vi "practica14RNA.vi"() -> ()   [LabVIEW 2016]
panel:
  out "XY Graph 2":cluster{dbl[], dbl[]}[](graph)
  out "axon":dbl
  in  "B":dbl
  in  "W2":dbl
  in  "W1":dbl
  in  "X2":dbl
  in  "X1":dbl
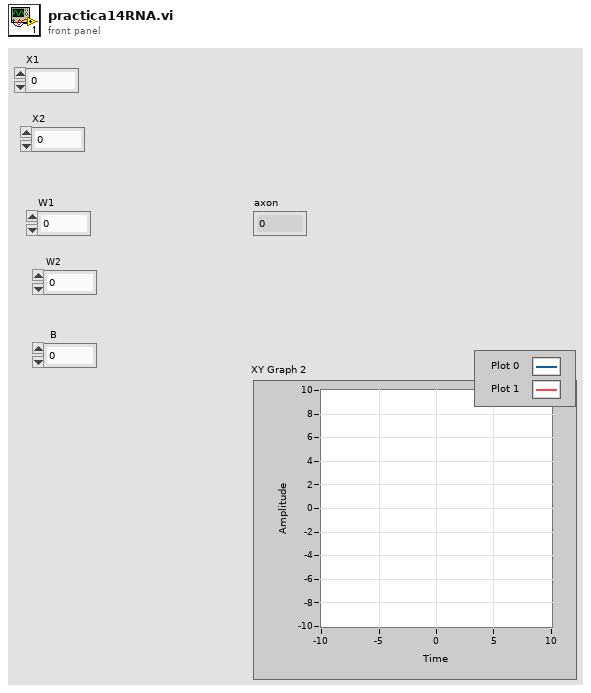
[diagram p1: front panel]
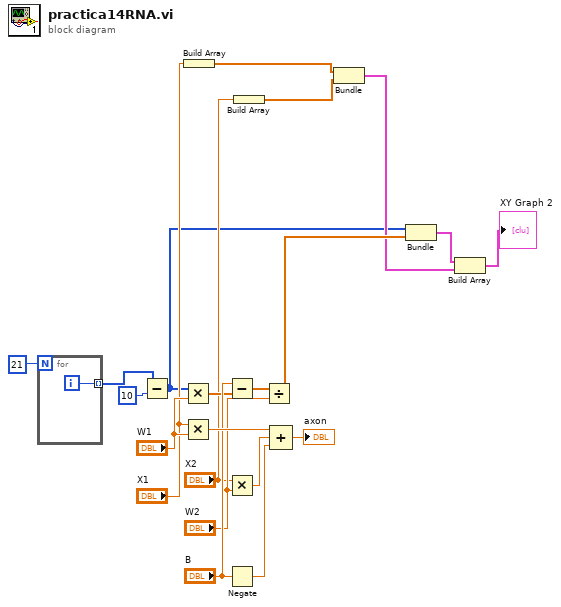
[diagram p0: block diagram]
diagram:
  n1 = for {
    N: 21 -> [_]
    tunnel: [w22] -> w2 mode=indexing
    i -> [w22]
  }
  n2 = Subtract(x=w2, y=10) -> (x-y=w1:i32[])
  n3 = Multiply(x=w1, y="W1") -> (x*y=w13:dbl[])
  n4 = Multiply(x="X1", y="W1") -> (x*y=w21:dbl)
  n5 = Build Array("X1") -> (w7:dbl[])
  n6 = Subtract(x="B", y=w13) -> (x-y=w12:dbl[])
  n7 = Multiply(x="X2", y="W2") -> (x*y=w20:dbl)
  n8 = Negate(x="B") -> (-x=w19:dbl)
  n9 = Build Array("X2") -> (w6:dbl[])
  n10 = Divide(x=w12, y="W2") -> (x/y=w11:dbl[])
  n11 = Compound Arithmetic op=ADD(w21, w20, w19) -> (→"axon":dbl)
  n12 = Bundle(w7, w6) -> (w4:cluster{dbl[], dbl[]})  [unwired: 1 in]
  n13 = Bundle(w1, w11) -> (w5:cluster{i32[], dbl[]})  [unwired: 1 in]
  n14 = Build Array(w5, w4) -> (→"XY Graph 2":cluster{dbl[], dbl[]}[])
